vi "AnalyzeWholeSignal.vi"() -> ()   [LabVIEW 2019]
uses:
  VibrationDiagnosisDesktopApp/mainVIs/DialogsVIs/AnalysisSettings.ctl
  MobileAnalyzer/mainVIs/analyzeAccelerationDataVIs/calculateFaultIndicatorsVIs/Thresholds.ctl
  MobileAnalyzer/mainVIs/analyzeAccelerationDataVIs/calculateFaultIndicatorsVIs/FaultParameter.ctl
  MobileAnalyzer/mainVIs/aquireAccelerationDataVIs/Accelerometer.ctl
  <vilib>/Analysis/5stat.llb/RMS (DBL).vi
  <vilib>/measure/madcrms.llb/Basic Averaged DC-RMS for 1 Chan.vi
  <vilib>/measure/madcrms.llb/Basic Averaged DC-RMS for N Chan.vi
  <vilib>/Analysis/NI_AALPro.lvlib
  <vilib>/measure/NI_MAPro.lvlib
panel:
  out "RMS values":dbl[][](array[numeric])
  out "DC values":dbl[][](array[numeric])
  in  "czułości [V/g]":dbl[][](array[numeric])=[[1.0, 1.0], [1.0, 1.0], [1.0, 1.0]]
  out "Rotational speed [RPM] 2":dbl format="%0.2f"
  out "rzędy 2":T1(graph)
  in  "sciezka 2":path
  out "FFT 2":cluster{"f0":dbl, "df":dbl, "real part":dbl[]}[](graph)
  out "rzędy":T1(graph)
  out "FFT":cluster{"f0":dbl, "df":dbl, "real part":dbl[]}[](graph)
  in  "AnalysisSettings":T2={"Fault Thresholds"={"Parameters labels"=[], "Parameters thresholds"=[], "Freqs and thresholds"=[], "Orders and thresholds"=[]}, "Analysis series name"="Analiza", "Save data analysis?"=TRUE, "F-Band Size"=20, "OrderAnalysis?"=TRUE, "Accelerometer"=enum."MMA7351", "fs [Hz]"=5120.0, "Pulse per revolution"=4, "FFT-Parameters"={"averaging mode"=enum."RMS averaging", "weighting mode"=enum."Linear", "number of averages"=1000}, "O-WindowPowerSpectrum"=1, "O-SpectrumAveraging"=enum."RMS averaging", "O-MaxOrder"=32.0, "O-Resolution"=0.1, "O-BandSize"=0.0, "FrameLength [s]"=1.0, "Aq.FrameLength [ms]"=1000, "FilterOrder"=32, "Sensitivity [V/g]"=[1.0, 1.0, 1.0]}
  out "tacho":waveform(dbl)(graph)
  out "acc":waveform(dbl)[](graph)
  in  "sciezka":path
  out "Rotational speed [RPM]":dbl format="%0.2f"
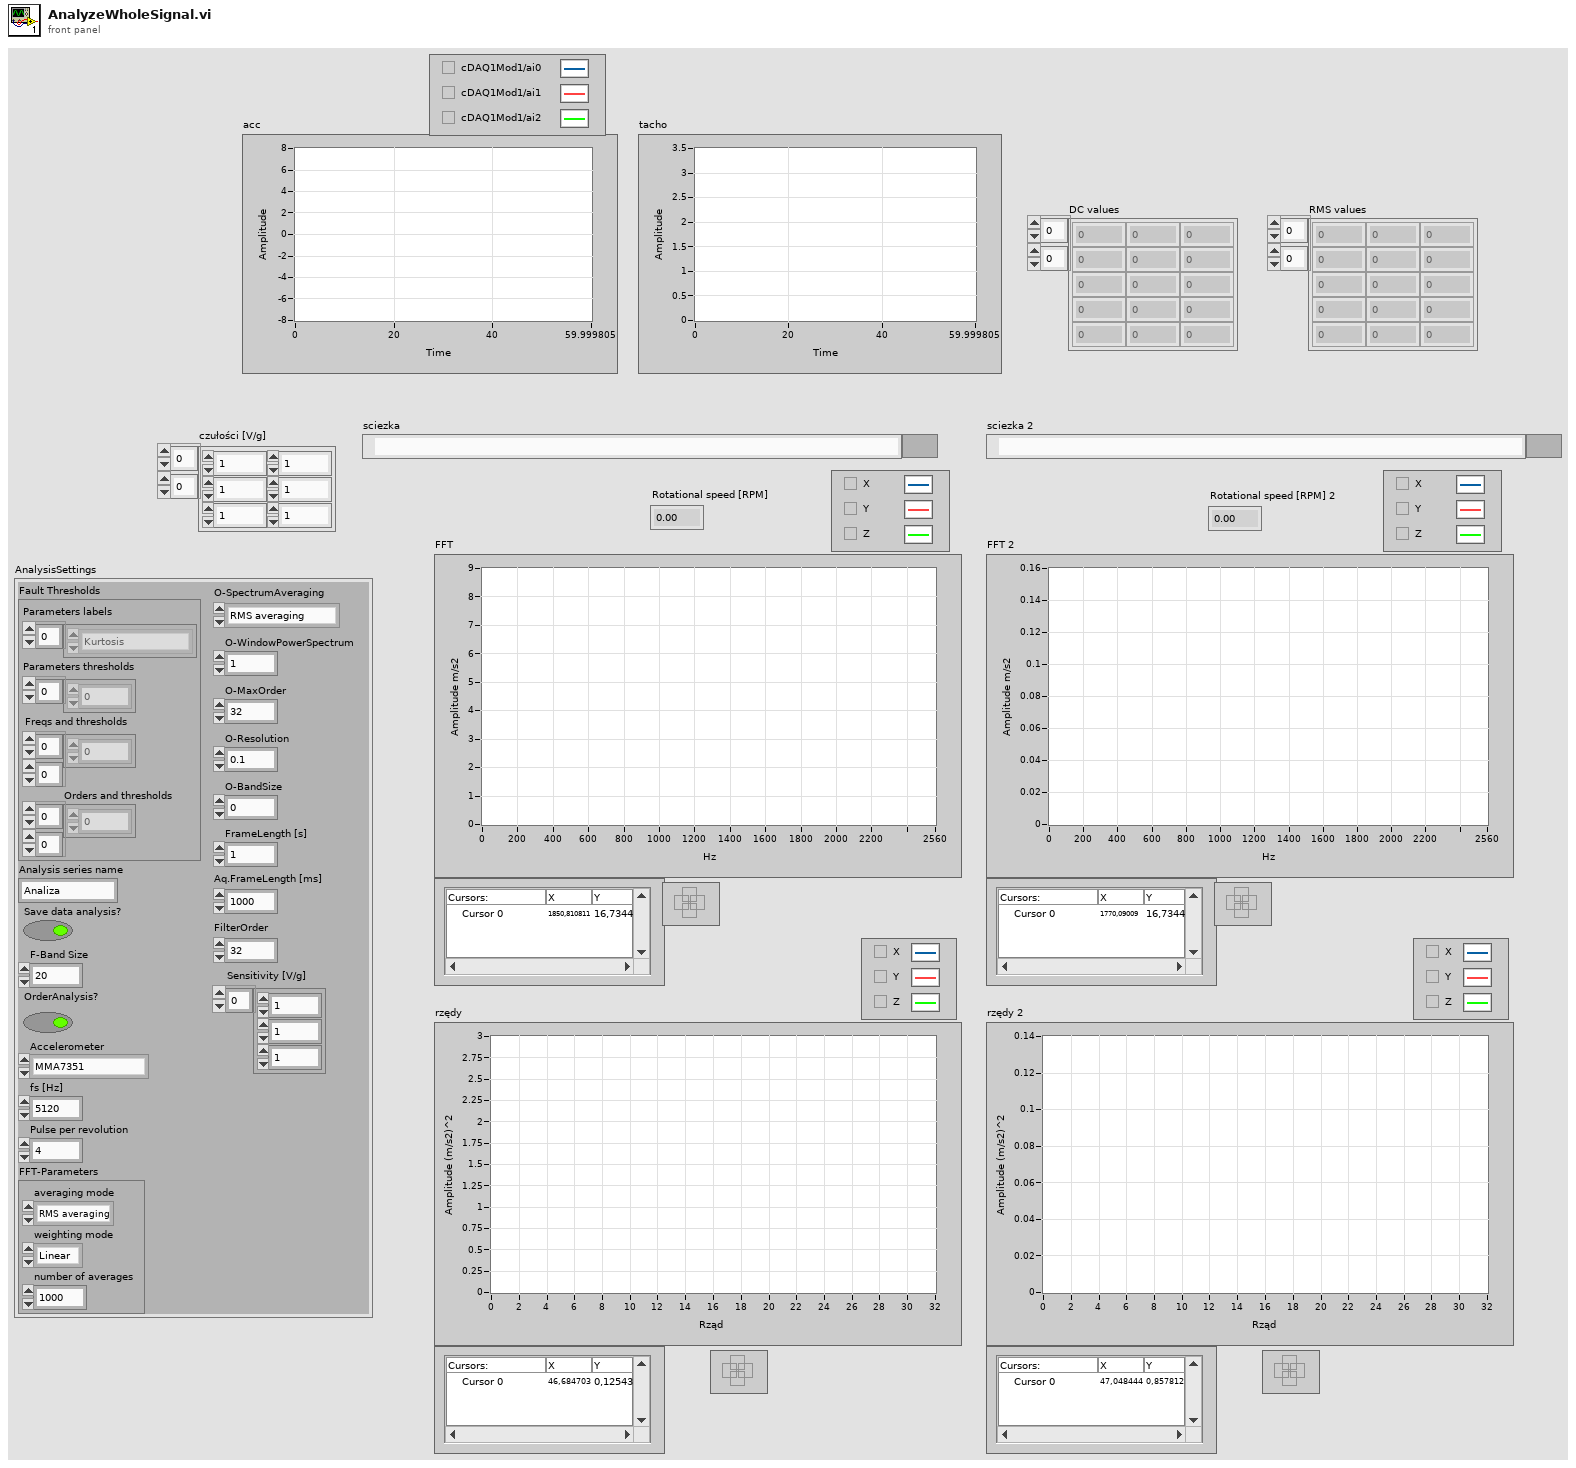
[diagram p1: front panel]
types:
  T1 = cluster{"order 0":dbl, "delta order":dbl, "magnitude":dbl[]}[]
  T2 = typedef "AnalysisSettings.ctl" = cluster{"Fault Thresholds":T3, "Analysis series name":string, "Save data analysis?":bool, "F-Band Size":i32, "OrderAnalysis?":bool, "Accelerometer":T5, "fs [Hz]":dbl, "Pulse per revolution":u16, "FFT-Parameters":cluster{"averaging mode":enum16{"No averaging", "Vector averaging", "RMS averaging", "Peak hold"}, "weighting mode":enum16{"Linear", "Exponential"}, "number of averages":u32}, "O-WindowPowerSpectrum":u32, "O-SpectrumAveraging":enum16{"No averaging", "Vector averaging", "RMS averaging", "Peak hold"}, "O-MaxOrder":dbl, "O-Resolution":dbl, "O-BandSize":dbl, "FrameLength [s]":dbl, "Aq.FrameLength [ms]":i64, "FilterOrder":i32, "Sensitivity [V/g]":dbl[]}
  T3 = typedef "Thresholds.ctl" = cluster{"Parameters labels":T4[], "Parameters thresholds":dbl[], "Freqs and thresholds":dbl[][], "Orders and thresholds":dbl[][]}
  T4 = typedef "FaultParameter.ctl" = enum16{"Kurtosis", "RMS", "Crest factor"}
  T5 = typedef "Accelerometer.ctl" = enum16{"None", "MPU6050", "MMA7351"}
  T6 = enum16{"open", "open or create", "create or replace", "create", "open (read-only)"}
  T7 = typedef "AccelerationDataFrames.ctl" = cluster{"AccelerationData":waveform(dbl)[], "Amplitudes":cluster{"f0":dbl, "df":dbl, "real part":dbl[]}[], "Phases":cluster{"f0":dbl, "df":dbl, "imaginary part":dbl[]}[]}
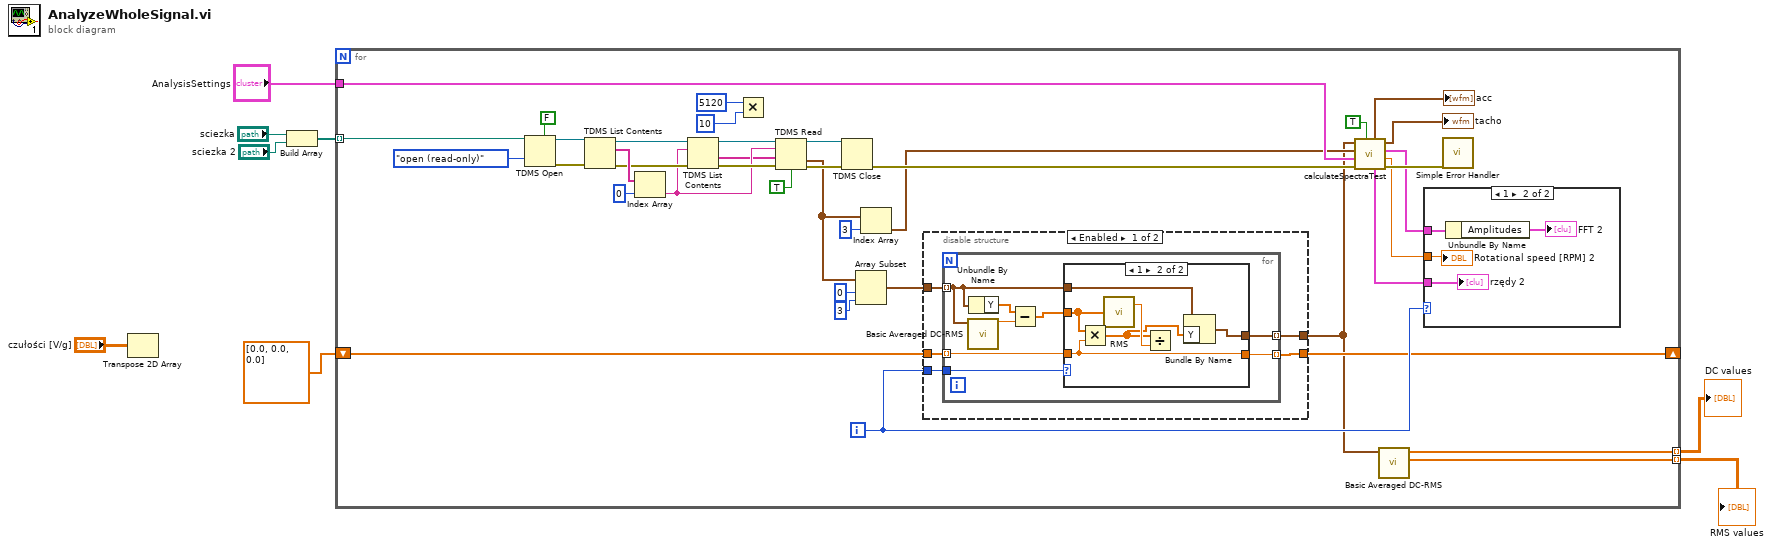
[diagram p0: block diagram]
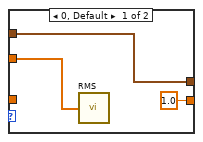
[diagram p2: hidden frame]
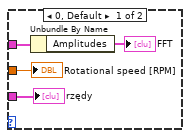
[diagram p4: hidden frame]
diagram:
  n1 = Transpose 2D Array(2D array="czułości [V/g]") -> ()  [unwired: 1 out]
  n2 = Build Array("sciezka", "sciezka 2") -> (w7:path[])
  n3 = for {
    tunnel: w7 -> [w45] mode=indexing
    tunnel: "AnalysisSettings" -> [w23]
    shift-right: [w15] -> _
    shift-left: dbl[] [0.0, 0.0, 0.0] ("czułości [V/g]") -> [w17]
    tunnel: [w11] -> w2 mode=indexing
    tunnel: [w10] -> w1 mode=indexing
    i -> [w16]
    n4 = TDMS Open(5:FALSE ("create index file? (T)"), 10:T6."open (read-only)" ("operation (0:open)"), 11:w45) -> (0:w34:errorcluster, 3:w35:refnum<k34>)  [unwired: 4 in]
    n5 = TDMS List Contents(4:w34, 7:w35) -> (0:w39:errorcluster, 2:w43:string[], 3:w41:refnum<k34>)  [unwired: 1 in, 1 out]
    n6 = Index Array(array=w43, index=0) -> (element=w37:string)
    n7 = TDMS List Contents(4:w39, 6:w37, 7:w41) -> (0:w38:errorcluster, 1:w36:string[], 3:w40:refnum<k34>)  [unwired: 1 out]
    n8 = Multiply(x=i64 5120 ("count (-1: all)"), y=i64 10) -> ()  [unwired: 1 out]
    n9 = TDMS Read(0:w40, 5:w37, 7:w36, 11:w38, 13:TRUE ("return channels in file order? (F)")) -> (4:w33:refnum<k34>, 10:w22:waveform(dbl)[], 15:w32:errorcluster)  [unwired: 3 in, 3 out]
    n10 = TDMS Close(8:w32, 11:w33) -> (0:w28:errorcluster)  [unwired: 1 out]
    n11 = Array Subset(array=w22, index=0, length=3) -> (w12:waveform(dbl)[])
    n12 = Index Array(array=w22, index=3) -> (element=w21:waveform(dbl))
    n13 = disable-structure shown="Enabled" {
      disable-tunnel: [w52 w71] -> w9
      disable-tunnel: w17 -> [w51 w70]
      disable-tunnel: w16 -> [w50 _]
      disable-tunnel: [w49 w70] -> w15
      disable-tunnel: w12 -> [w48 w71]
      frame Enabled {
        n14 = for {
          tunnel: w48 -> [w56] mode=indexing
          tunnel: [w60] -> w52 mode=indexing
          tunnel: w51 -> [w57] mode=indexing
          tunnel: w50 -> [w59]
          tunnel: [w58] -> w49 mode=indexing
          n15 = call-poly <vilib>:"Basic Averaged DC-RMS.vi"("signal in"=w56) -> ("DC value"=w55:dbl)  [unwired: 7 in, 3 out]
          n16 = Unbundle By Name(w56) -> ("Y"=w54:dbl[])
          n17 = Subtract(x=w54, y=w55) -> (x-y=w53:dbl[])
          n18 = case shown="1" w59 {
            tunnel: w56 -> [w63 w69]
            tunnel: [w63 w68] -> w60
            tunnel: w53 -> [w62 w66]
            tunnel: [1.0 ("Numeric") w67] -> w58
            tunnel: w57 -> [_ w67]
            frame 0, Default {
              n19 = call-poly <vilib>:"RMS.vi"("X"=w62) -> ()  [unwired: 2 out]
            }
            frame 1 {
              n20 = Multiply(x=w66, y=w67) -> (x*y=w64:dbl[])
              n21 = call-poly <vilib>:"RMS.vi"("X"=w66) -> ("rms value"=w65:dbl)  [unwired: 1 out]
              n22 = Divide(x=w64, y=w65) -> ()  [unwired: 1 out]
              n23 = Bundle By Name(cluster=w69, "Y"=w64) -> (w68:waveform(dbl))
            }
          }
        }
      }
      frame Disabled {
      }
    }
    n24 = call "calculateSpectraTest.vi"("Reset?"=TRUE, "ErrorIn"=w28, "AnalysisSettings"=w23, "Tacho signal In"=w21, "AccelerationDataIn"=w9) -> ("ErrorOut"=w27:errorcluster, "Rotational speed [RPM]"=w26:dbl, "AccelerationDataFrames"=w25:T7, "Tacho signal out"=→"tacho":waveform(dbl), "order power spectra"=w24:T1, "AccelerationDataOut"=→"acc":waveform(dbl)[])  [unwired: 1 out]
    n25 = call-poly <vilib>:"Basic Averaged DC-RMS.vi"("signals in"=w9) -> ("RMS values"=w10:dbl[], "DC values"=w11:dbl[])  [unwired: 7 in, 2 out]
    n26 = case shown="1" w16 {
      tunnel: w26 -> [w75 w76]
      tunnel: w25 -> [w73 w78]
      tunnel: w24 -> [w72 w79]
      frame 0, Default {
        n27 = Unbundle By Name(w73) -> ("Amplitudes"=→"FFT":cluster{"f0":dbl, "df":dbl, "real part":dbl[]}[])
        "Rotational speed [RPM]" <- w75
        "rzędy" <- w72
      }
      frame 1 {
        n28 = Unbundle By Name(w78) -> ("Amplitudes"=→"FFT 2":cluster{"f0":dbl, "df":dbl, "real part":dbl[]}[])
        "rzędy 2" <- w79
        "Rotational speed [RPM] 2" <- w76
      }
    }
    n29 = call <vilib>:"Simple Error Handler.vi"("error in (no error)"=w27) -> ()  [unwired: 4 in, 5 out]
  }
  "DC values" <- w2
  "RMS values" <- w1
